vi "command engine get time delta.vi"(8 "error in (no error)":errorcluster, 9 "State Variables in":T13, 10 "Parameters":T2 {"Compiled"."External Channels"."Channels" format="%.0x"; "Compiled"."External Channels"."Triggers" format="%.0x"}, 11 "Global Variables":T1) -> (0 "error out":errorcluster, 1 "State Variables out":T13, 2 "Parameters out":T2 {"Compiled"."External Channels"."Channels" format="%.0x"; "Compiled"."External Channels"."Triggers" format="%.0x"}, 3 "Global Variables out":T1)   [LabVIEW 2015, in "Instrument Addon Engine.lvlib"]
uses:
  Instrument Addon Engine.lvlib
  Types/command engine global variables.ctl
  <vilib>/NI/AMC/Message Queue.ctl
  <vilib>/NI/AMC/Message.ctl
  <vilib>/NI/Tools/Keyed Array/KeyedArray.ctl
  Types/Commands RT Configuration Cluster.ctl
  Protocols.lvlibp/Protocol Parent/Protocol Parent.lvclass
  Shared/Types/Compiled Settings.ctl
  Shared/Types/Command Parameters.ctl
  Shared/Types/Linked Channel Cluster.ctl
  Shared/Types/Response RT Configuration Cluster.ctl
  Shared/Types/Response Parameters.ctl
  Shared/Types/Response Wait Type.ctl
  Shared/Types/Message Parameters.ctl
  Shared/Types/Message Generation Type.ctl
  Shared/Types/External Trigger Refs.ctl
  <vilib>/NI Veristand/Custom Device API/Data Reference.ctl
  Protections.lvlibp/Parent Protection/Protection.lvclass
  Types/Engine State Variables.ctl
  <vilib>/NI/NIVS Inline Async API/_VS Inline Async API/Process/Process.lvclass
  <vilib>/NI/NIVS Addon Network Comm/Engine/VeriStand Comm.lvclass
  <vilib>/NI/NIVS Inline Async API/_Data Access Engine/Access Type Classes/Write/Write.lvclass
  <vilib>/NI/NIVS Inline Async API/_Data Access Engine/Access Type Classes/Read/Read.lvclass
  <vilib>/NI/NIVS Inline Async API/_Data Access Engine/Access Type Classes/ReadWrite/ReadWrite.lvclass
  <vilib>/NI/Tools/Keyed Array/Tools_KeyedArray.lvlib
  <vilib>/NI/AMC/AMC.lvlib
  Shared/Instrument Addon Shared.lvlib
  <vilib>/NI VeriStand/Custom Device API/Custom Device API.lvlib
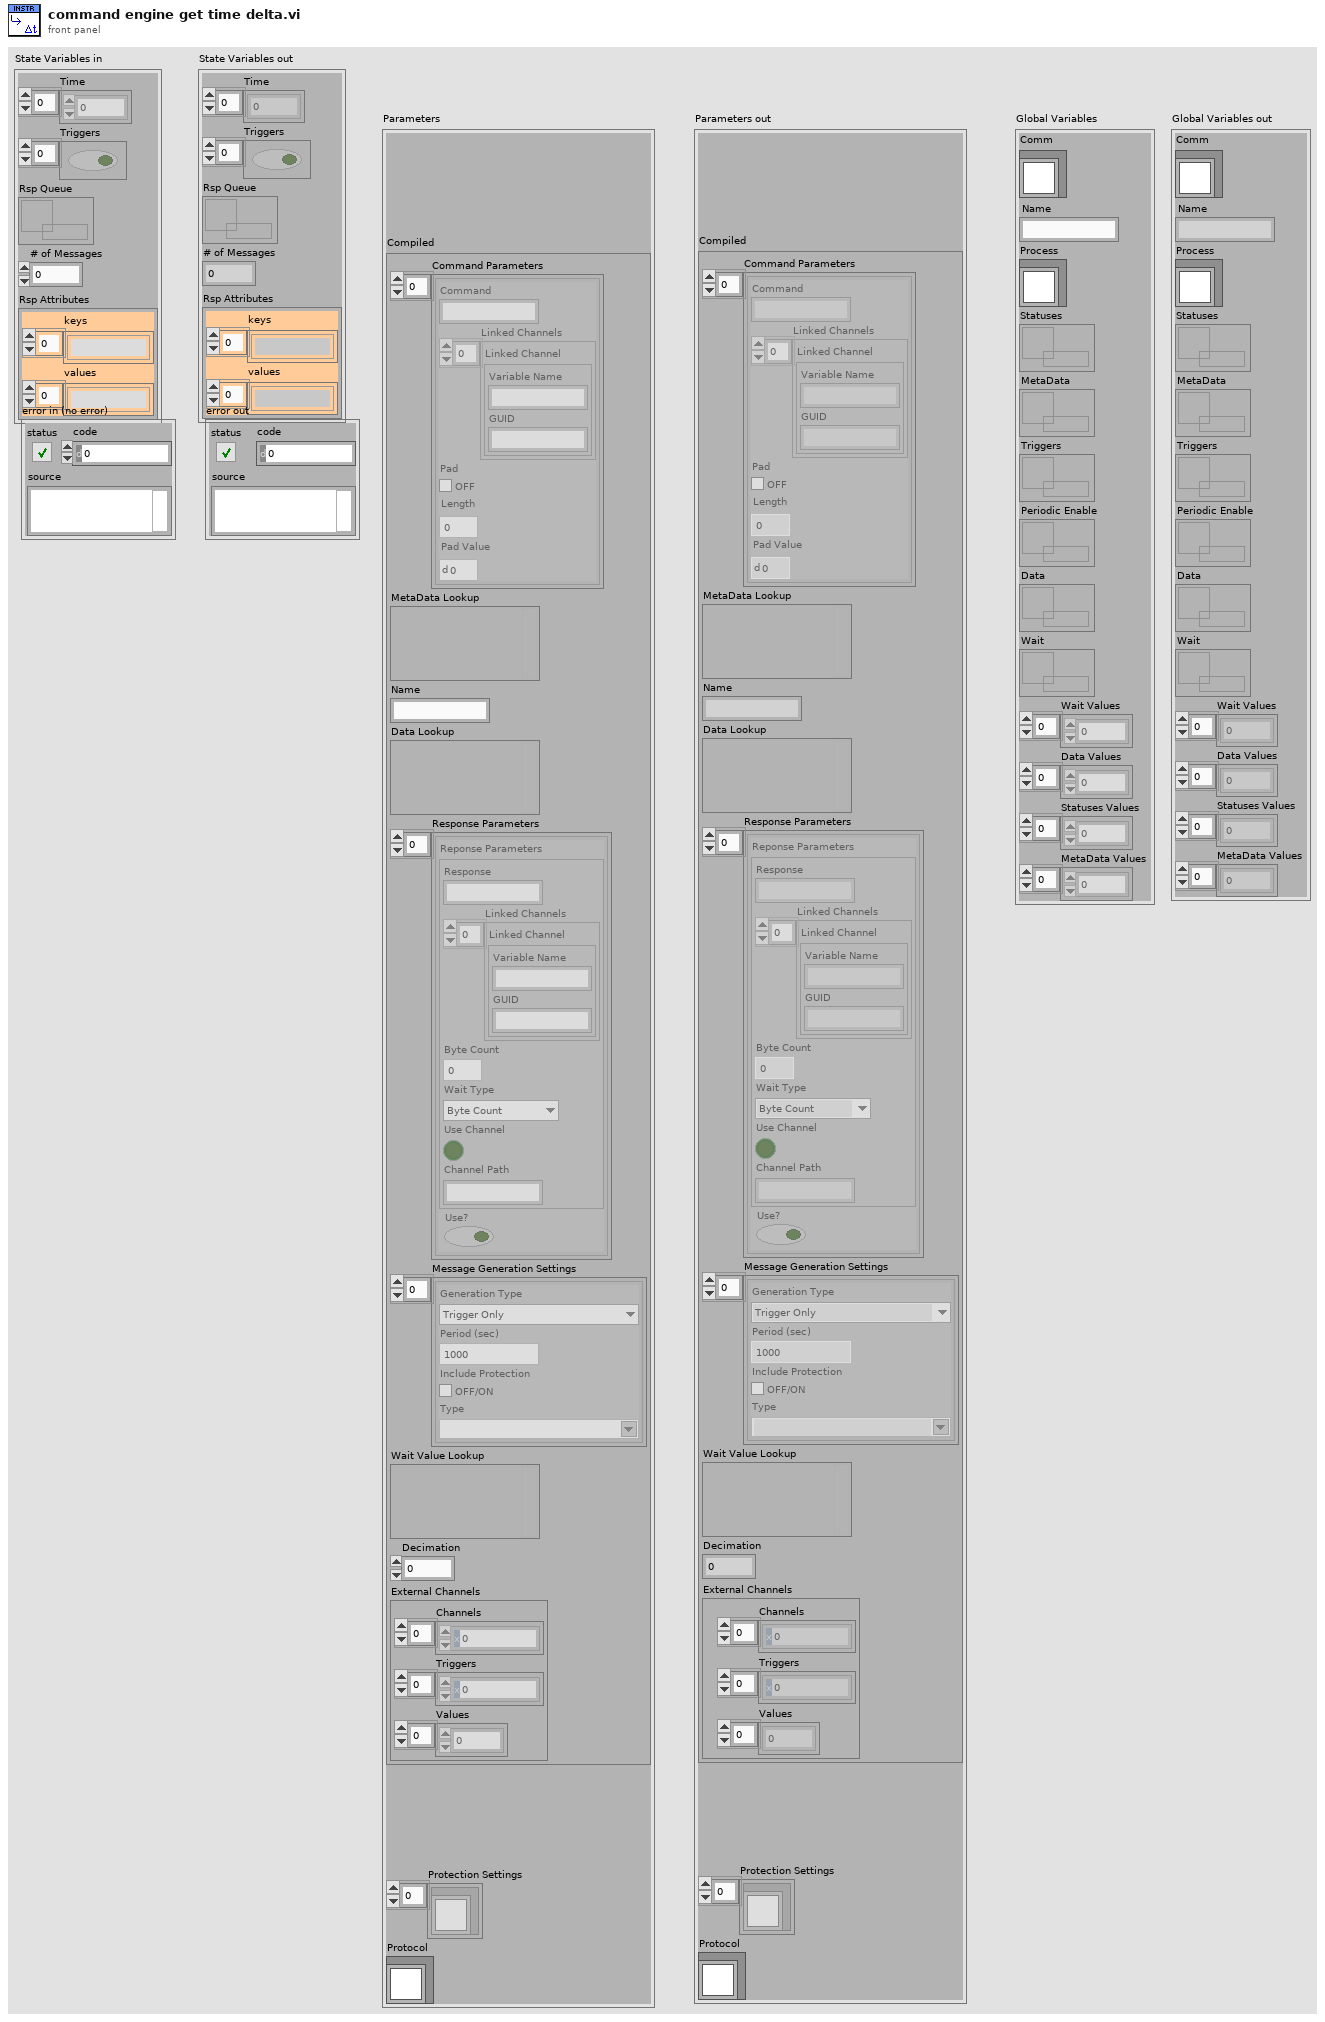
[diagram p1: front panel]
types:
  T1 = typedef "Instrument Addon Engine.lvlib/Engine State Variables.ctl" = cluster{"Comm":refnum<class "VeriStand Comm.lvclass">, "Name":string, "Process":refnum<class "Process.lvclass">, "Statuses":refnum<data-value>, "MetaData":refnum<data-value>, "Triggers":refnum<data-value>, "Periodic Enable":refnum<data-value>, "Data":refnum<data-value>, "Wait":refnum<data-value>, "Wait Values":dbl[], "Data Values":dbl[], "Statuses Values":dbl[], "MetaData Values":dbl[]}
  T2 = typedef "Instrument Addon Engine.lvlib/Commands RT Configuration Cluster.ctl" = cluster{"Compiled":T3, "Protection Settings":refnum<class "Protection.lvclass">[], "Protocol":refnum<class "Protocol Parent.lvclass">}
  T3 = typedef "Instrument Addon Shared.lvlib/Compiled Settings.ctl" = cluster{"Command Parameters":T4[], "MetaData Lookup":variant, "Name":string, "Data Lookup":variant, "Response Parameters":T6[], "Message Generation Settings":T9[], "Wait Value Lookup":variant, "Decimation":u32, "External Channels":T11}
  T4 = typedef "Instrument Addon Shared.lvlib/Command Parameters.ctl" = cluster{"Command":string, "Linked Channels":T5[], "Pad":bool, "Length":u32, "Pad Value":u8}
  T5 = typedef "Instrument Addon Shared.lvlib/Linked Channel Cluster.ctl" = cluster{"Variable Name":string, "GUID":string}
  T6 = typedef "Instrument Addon Shared.lvlib/Response RT Configuration Cluster.ctl" = cluster{"Reponse Parameters":T7, "Use?":bool}
  T7 = typedef "Instrument Addon Shared.lvlib/Response Parameters.ctl" = cluster{"Response":string, "Linked Channels":T5[], "Type Value":dbl, "Wait Type":T8, "Use Channel":bool, "Channel Path":string}
  T8 = typedef "Instrument Addon Shared.lvlib/Response Wait Type.ctl" = enum16{"Byte Count", "Wait sec"}
  T9 = typedef "Instrument Addon Shared.lvlib/Message Parameters.ctl" = cluster{"Generation Type":T10, "Period":dbl, "Include Protection":bool, "Type":string}
  T10 = typedef "Instrument Addon Shared.lvlib/Message Generation Type.ctl" = enum16{"Trigger Only", "Periodic & Trigger"}
  T11 = typedef "Instrument Addon Shared.lvlib/External Trigger Refs.ctl" = cluster{"Channels":T12[], "Triggers":T12[], "Values":dbl[]}
  T12 = typedef "Custom Device API.lvlib/Data Reference.ctl" = i32
  T13 = typedef "Instrument Addon Engine.lvlib/command engine global variables.ctl" = cluster{"Time":u32[], "Triggers":bool[], "Rsp Queue":T14, "# of Messages":i32, "Rsp Attributes":T15}
  T14 = typedef "AMC.lvlib/Message Queue.ctl" = refnum<queue>
  T15 = typedef "Tools_KeyedArray.lvlib/KeyedArray.ctl" = cluster{"keys":string[], "values":string[]}
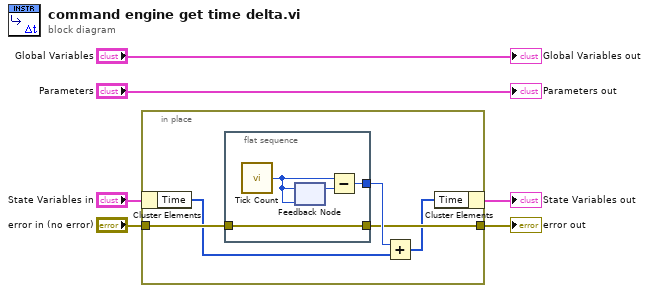
[diagram p0: block diagram]
diagram:
  n1 = in-place {
    in-place-border: "error in (no error)" -> [w11]
    in-place-border: [w9] -> w4
    n2 = in-place-cluster #1("State Variables in") -> ("Time"=w8:u32[])
    n3 = flat-sequence {
      tunnel: [w15] -> w9
      tunnel: w11 -> [w15]
      tunnel: [w12] -> w10
      frame #0 {
        n4 = call "Tick Count"() -> ("Tick Count(uSec)"=w13:u32)
        n5 = feedback-in #2(w13) -> ()
        n6 = feedback #2(w13) -> (w14:u32)
        n7 = Subtract(x=w13, y=w14) -> (x-y=w12:u32)
      }
    }
    n8 = Add(x=w10, y=w8) -> (x+y=w7:u32[])
    n9 = in-place-cluster #1("Time"=w7) -> (→"State Variables out":T13)
  }
  "error out" <- w4
  "Global Variables out" <- "Global Variables"
  "Parameters out" <- "Parameters"
